vi "macro_Cmd_FindFollowRamseteSimpleExecute.vi"() -> ()   [LabVIEW 2019, in "PathPlanner24.lvlib"]
uses:
  PathPlanner24.lvlib
  <vilib>/Rock Robotics/WPI/ThirdParty/JAS_Junk/TrajLib/Trajectory_Library.lvlib
  <vilib>/Rock Robotics/WPI/ThirdParty/JAS_Junk/TrajLib/TypeDef/CHASSIS_SPEEDS.ctl
  <vilib>/Rock Robotics/WPI/ThirdParty/JAS_Junk/TrajLib/TypeDef/ROTATION2D.ctl
  <vilib>/Rock Robotics/WPI/ThirdParty/JAS_Junk/TrajLib/TypeDef/TRANSLATION2D.ctl
  <vilib>/Rock Robotics/WPI/ThirdParty/JAS_Junk/TrajLib/TypeDef/POSE2D.ctl
panel:
  in  "Target Pose M":T1={"TRANSLATION"={"X"=0.0, "Y"=0.0}, "ROTATION"={"VALUE"=0.0, "COS"=1.0, "SIN"=0.0}} {"ROTATION"."SIN" format="%13.4f"; "ROTATION"."COS" format="%13.4f"; "ROTATION"."VALUE" format="%13.4f"; "TRANSLATION"."Y" format="%14.3f"; "TRANSLATION"."X" format="%14.3f"}
  out "Complete":bool
  in  "CurrentChassisSpeeds 2":T4 {"vOmega" format="%10.3f"; "vY" format="%10.3f"; "vX" format="%10.3f"}
  out "Right Speed Dmd M/S":dbl
  out "Left Speed Dmd M/S":dbl
  in  "Reset 2":bool
  in  "currentPose 2":T1={"TRANSLATION"={"X"=0.0, "Y"=0.0}, "ROTATION"={"VALUE"=0.0, "COS"=1.0, "SIN"=0.0}} {"ROTATION"."SIN" format="%13.4f"; "ROTATION"."COS" format="%13.4f"; "ROTATION"."VALUE" format="%13.4f"; "TRANSLATION"."Y" format="%14.3f"; "TRANSLATION"."X" format="%14.3f"}
  out "Position Error M":dbl
  out "At Reference":bool
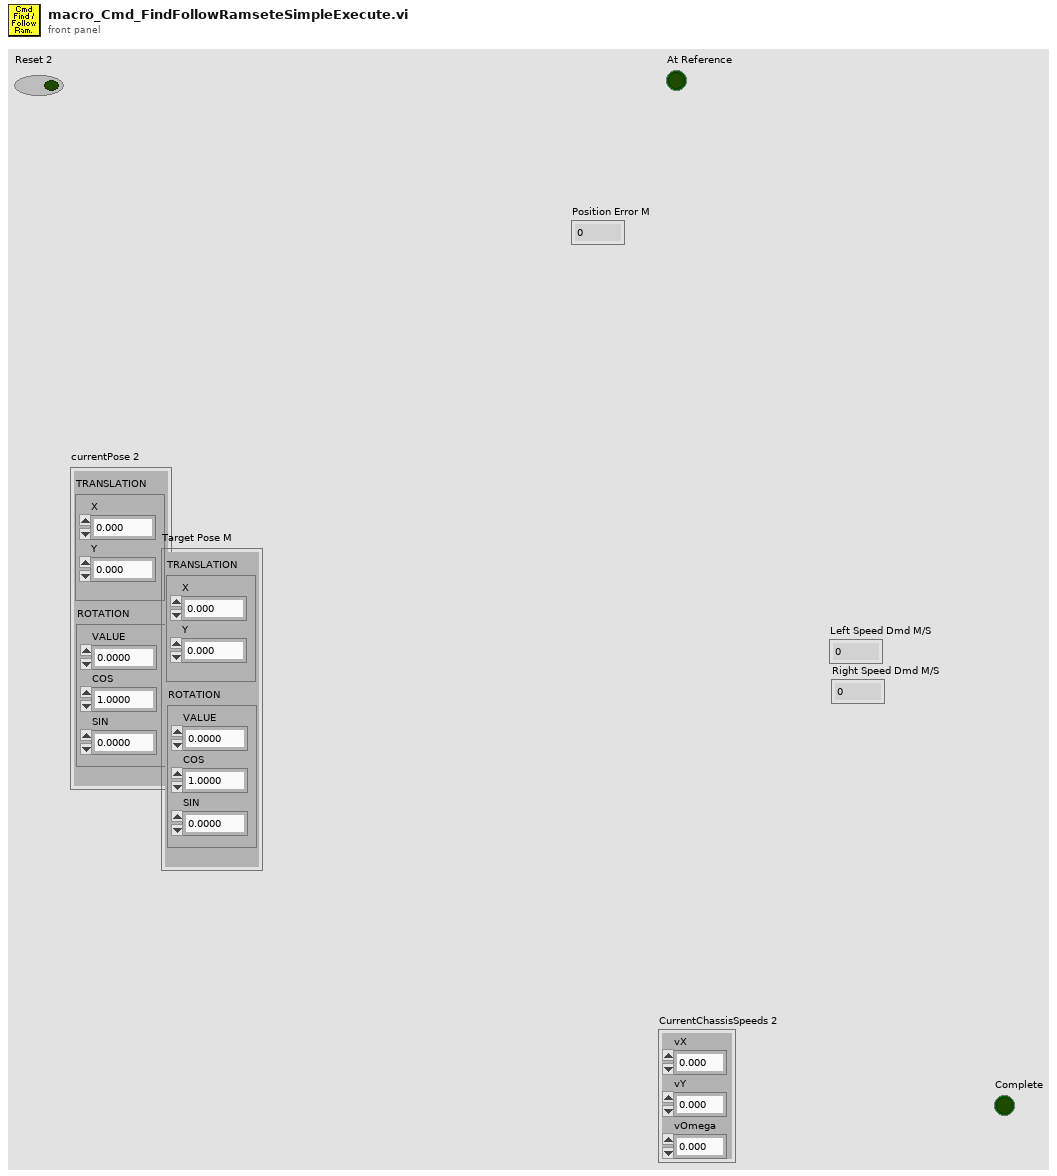
[diagram p1: front panel]
types:
  T1 = typedef "Trajectory_Library.lvlib/POSE2D.ctl" = cluster{"TRANSLATION":T2, "ROTATION":T3}
  T2 = typedef "Trajectory_Library.lvlib/TRANSLATION2D.ctl" = cluster{"X":dbl, "Y":dbl}
  T3 = typedef "Trajectory_Library.lvlib/ROTATION2D.ctl" = cluster{"VALUE":dbl, "COS":dbl, "SIN":dbl}
  T4 = typedef "Trajectory_Library.lvlib/CHASSIS_SPEEDS.ctl" = cluster{"vX":dbl, "vY":dbl, "vOmega":dbl}
  T5 = typedef "PathPlanner24.lvlib/PathPlannerPathConstraints.ctl" = cluster{"MaxVelocityMps;":dbl, "MaxAccelerationMpsSq;":dbl, "MaxAngularVelRadPsEc;":dbl, "MaxAngularAccRadPSecSq":dbl, "Exists":bool, "Unlimited":bool, "NominalVoltageVolts":dbl}
  T6 = typedef "Trajectory_Library.lvlib/RAMSETE_EXE_TUNING.ctl" = cluster{"B":dbl, "Zeta":dbl, "X Tolerance M":dbl, "Y Tolerance M":dbl, "Heading Tolerance RAD":dbl, "Track Width M":dbl, "Max Speed M/S":dbl}
  T7 = typedef "PathPlanner24.lvlib/PathPlannerCmdFollowRamConfig.ctl" = cluster{"ControlPastEnd_Sec":dbl, "Trigger Events":bool, "RAMSETE_EXE_TUNING SI":T6}
  T8 = typedef "PathPlanner24.lvlib/PathPlannerCmdFindConfig.ctl" = cluster{"Goal Position":T2, "GoalEndState":T9, "PathPlannerPathConstraints":T5, "Rotation Delay Distance M":dbl}
  T9 = typedef "PathPlanner24.lvlib/PathPlannerGoalEndState.ctl" = cluster{"VelocityMPS":dbl, "Rotation":T3}
  T10 = cluster{"Left Speed Dmd M/S":dbl, "Right Speed Dmd M/S":dbl}
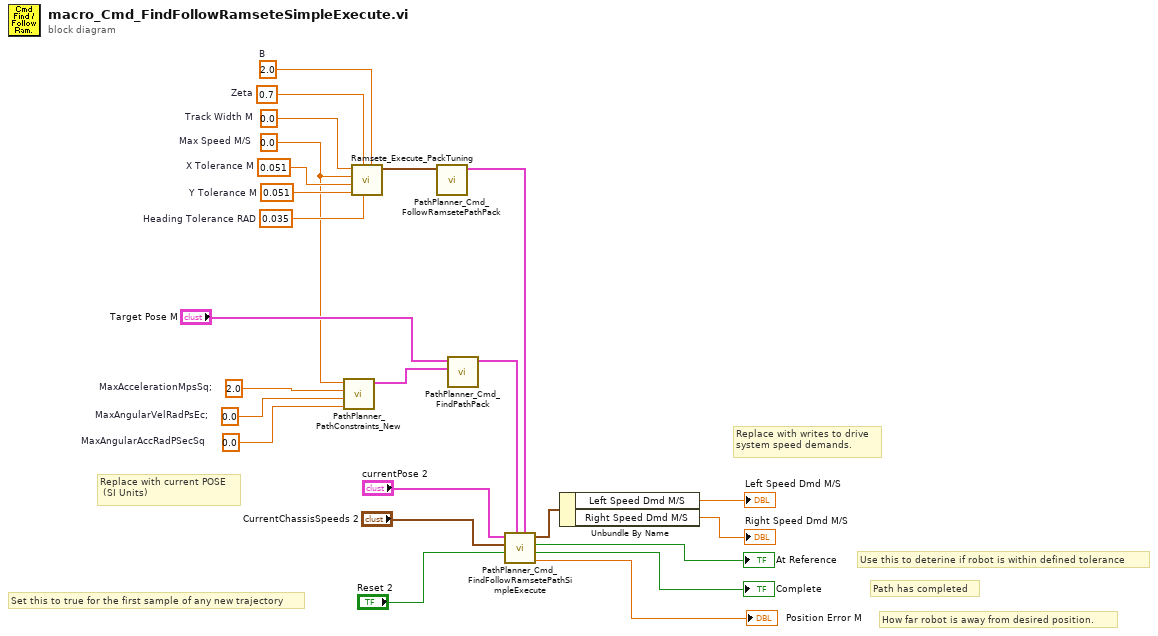
[diagram p0: block diagram]
diagram:
  w1 = 0.0  # MaxAngularAccRadPSecSq
  w2 = 0.0  # MaxAngularVelRadPsEc;
  w6 = 2.0  # MaxAccelerationMpsSq;
  w24 = 0.0  # Track Width M
  w3 = 0.0  # Max Speed M/S
  w23 = 0.051  # X Tolerance M
  w22 = 0.051  # Y Tolerance M
  w21 = 0.7  # Zeta
  w20 = 0.035  # Heading Tolerance RAD
  w19 = 2.0  # B
  # "Path has completed"
  # "Replace with writes to drive\nsystem speed demands."
  # "Replace with current POSE\n (SI Units)"
  # "How far robot is away from desired position."
  # "Use this to deterine if robot is within defined tolerance"
  # "Set this to true for the first sample of any new trajectory"
  n1 = call "PathPlanner_PathConstraints_New.vi"("MaxAngularAccRadPSecSq"=w1, "MaxAngularVelRadPsEc;"=w2, "MaxAccelerationMpsSq;"=w6, "MaxVelocityMps;"=w3) -> ("PathPlannerConstraints"=w5:T5)  [unwired: 7 in]
  n2 = call <vilib>:"Ramsete_Execute_PackTuning.vi"("B"=w19, "Heading Tolerance RAD"=w20, "Zeta"=w21, "Y Tolerance M"=w22, "X Tolerance M"=w23, "Max Speed M/S"=w3, "Track Width M"=w24) -> ("RAMSETE_EXE_TUNING"=w17:T6)  [unwired: 4 in]
  n3 = call "PathPlanner_Cmd_FollowRamsetePathPack.vi"("RAMSETE_EXE_TUNING"=w17) -> ("PathPlanner_Ctrl_RamDrvConfig"=w18:T7)  [unwired: 10 in]
  n4 = call "PathPlanner_Cmd_FindPathPack.vi"("PathPlannerPathConstraints"=w5, "Target Pose M"="Target Pose M") -> ("PathPlanner_Cmd_FindConfig"=w4:T8)  [unwired: 9 in]
  n5 = call "PathPlanner_Cmd_FindFollowRamsetePathSimpleExecute.vi"("PathPlanner_Cmd_FollowRamConfig"=w18, "PathPlanner_Cmd_FindConfig"=w4, "Reset"="Reset 2", "CurrentChassisSpeeds"="CurrentChassisSpeeds 2", "Current Pose SI"="currentPose 2") -> ("Position Error M"=→"Position Error M":dbl, "Complete"=→"Complete":bool, "At Reference"=→"At Reference":bool, "Left Right Speed Dmds"=w13:T10)  [unwired: 2 in, 1 out]
  n6 = Unbundle By Name(w13) -> ("Left Speed Dmd M/S"=→"Left Speed Dmd M/S":dbl, "Right Speed Dmd M/S"=→"Right Speed Dmd M/S":dbl)
